vi "Is Sub-Block Complete.vi"(11 "Block Upload Sub-Block Transfer in":refnum<class "Block Upload Sub-Block Transfer.lvclass">) -> (2 "Complete":bool, 3 "Block Upload Sub-Block Transfer out":refnum<class "Block Upload Sub-Block Transfer.lvclass">)   [LabVIEW 2020, in "CANopen.lvlib" / "SDO Manager.lvlib" / "Block Upload Sub-Block Transfer.lvclass"]
uses:
  Block Upload Sub-Block Transfer.lvclass
  D:/git/CANopen-LabVIEW/source/SDO Manager/SDO Manager/Block Upload Initiate Transfer/Block Upload Initiate Transfer.lvclass
  Block Upload Sub-Block Transfer.lvclass/Block Upload Sub-Block Transfer.ctl
  Block Upload Initiate Transfer/Block Upload Initiate Transfer.lvclass/Block Upload Initiate Transfer.ctl
  Block Upload Initiate Transfer/Block Upload Initiate Transfer.lvclass
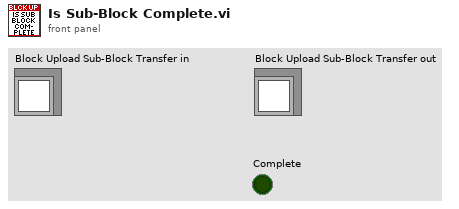
[diagram p1: front panel]
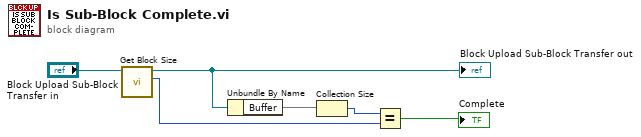
[diagram p0: block diagram]
diagram:
  n1 = call "Get Block Size.vi"("Block Upload Initiate in"="Block Upload Sub-Block Transfer in") -> ("Block Size"=w1:u8, "Block Upload Initiate out"=w4:refnum<class "Block Upload Sub-Block Transfer.lvclass">)  [unwired: 8 in, 1 out]
  "Block Upload Sub-Block Transfer out" <- w4
  n2 = Unbundle By Name(w4) -> ("Buffer"=w5:map{u8, u8[]})
  n3 = Collection Size(1:w5) -> (0:w2:i32)
  n4 = Equal?(x=w2, y=w1) -> (x = y?=→"Complete":bool)
